vi "ProdaNG.LogIn.vi"(8 "error in":errorcluster, 11 "ConnectionString":string) -> (0 "error out":errorcluster, 2 "User":string, 3 "dbHandle":i32)   [LabVIEW 2016]
doc: "This function offers the logon to an Oracle database and can be called in every Thread. In case that the DLL is running in a Shared Context, an existing connection to ORACLE will be terminated first and afterwards reconstructed! In the other case the connection is constructed and a new Handle is created. During the Login phase it is being tried repeatedly to establish the connection to the database. The number of retries is 5, each with 5 seconds standby time between the efforts. If a connection is not possible, this function returns afterwards with the responding Oracle error code.\n\nWhen the Login is successful, the above-quoted preferences will be read from the database. \nA successful connection to the database requires a correct definition of NET- respective Sqlnet-settings on the used Client.\nParameter:\nuser, password and database are the single parts of the syntax at the \nLogon with the Oracle database tools:\n\nUSERNAME/PASSWORD@DBNAME\n\nuser User account in the database\npassword Password of the database user account\ndatabase Service name or SID of the used database\n\n*handle is filled with the new handle, if the returncode=0.\n\nReturncodes:\n0 no error\n< 0 ORACLE error code. Because no valid handle was created, the function GetLastErrorMsg() cannot be used.\n1 Context is no longer available. In this case numContexts in InitProDll() should be increased."
uses:
  prodllNG.dll
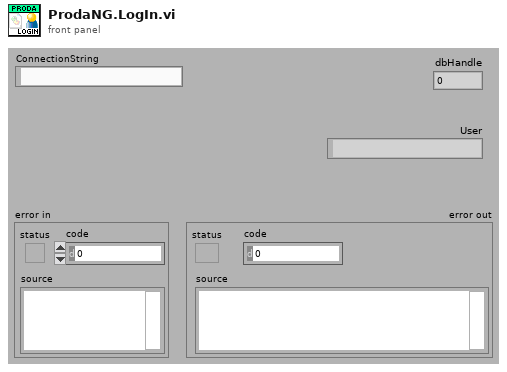
[diagram p1: front panel]
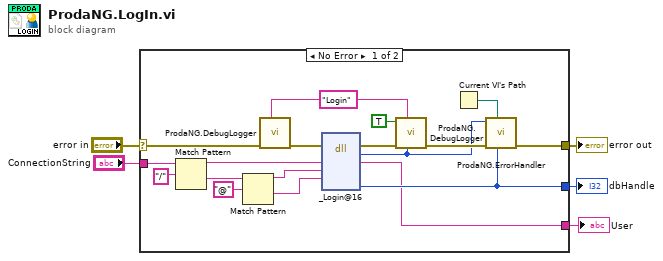
[diagram p0: block diagram]
diagram:
  n1 = case shown="No Error" "error in" {
    selector: "error in" -> [w18 w23]
    tunnel: [w22 w23] -> w4
    tunnel: [w14 _] -> w3
    tunnel: "ConnectionString" -> [w9 _]
    tunnel: [w6 _] -> w1
    frame No Error {
      w20 = "Login" ("cmd")
      n2 = Match Pattern(string=w9, regular expression="/") -> (before substring=w6:string, after substring=w12:string)  [unwired: 1 in, 2 out]
      n3 = Match Pattern(string=w12, regular expression="@") -> (before substring=w8:string, after substring=w7:string)  [unwired: 1 in, 2 out]
      n4 = call "ProdaNG.DebugLogger.vi"("cmd"=w20, "error in (no error)"=w18) -> ("error out"=w17:errorcluster)  [unwired: 9 in]
      n5 = dll-call lib="D:/Maszup/WABCO/SVN/LineTraceSystem/SOFTWARE/sources/Database/ProdaNG/prodllNG.dll" fn="_Login@16" ("ProDll.dll:Login")(error in=w17, "user"=w6, "password"=w8, "database"=w7) -> (error out=w16:errorcluster, w13:i32, "dbHandle"=w14:i32)  [unwired: 6 in, 1 out]
      n6 = call "ProdaNG.DebugLogger.vi"("return type"=w13, "cmd"=w20, "error in (no error)"=w16, "done? (F)"=TRUE) -> ("error out"=w15:errorcluster)  [unwired: 7 in]
      n7 = Current VI's Path() -> (path=w21:path)
      n8 = call "ProdaNG.ErrorHandler.vi"("dbHandleIn"=w14, "Path"=w21, "error in"=w15, "output_parameter"=w13) -> ("error out"=w22:errorcluster)  [unwired: 7 in]
    }
    frame Error {
    }
  }
  "error out" <- w4
  "dbHandle" <- w3
  "User" <- w1
